vi "open_browser_send_url.vi"() -> ()   [LabVIEW 2018]
doc: "This VI uses ActiveX to open IE in its own window and point it to the URL typed into the string control."
panel:
  in  "Enter a URL and run the VI":string="http://192.168.169.3"
  in  "SHDocVw.IWebBrowser2":refnum<k7>
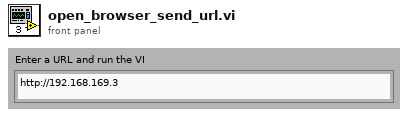
[diagram p1: front panel]
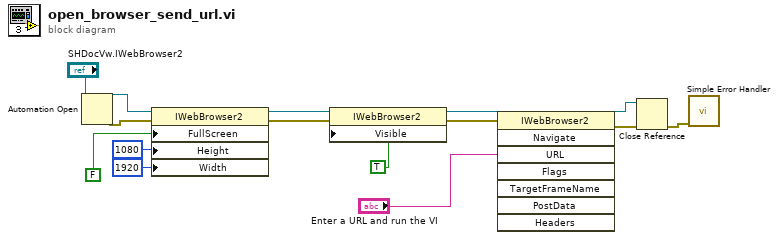
[diagram p0: block diagram]
diagram:
  n1 = Automation Open(Automation Refnum="SHDocVw.IWebBrowser2") -> (Automation Refnum=w15:refnum<k7>, error out=w14:errorcluster)  [unwired: 3 in]
  n2 = property class="IWebBrowser2"(reference=w15, error in=w14, "FullScreen"=FALSE, "Height"=1080, "Width"=1920) -> (reference out=w5:refnum<k7>, error out=w4:errorcluster)
  n3 = property class="IWebBrowser2"(reference=w5, error in=w4, "Visible"=TRUE) -> (reference out=w11:refnum<k7>, error out=w12:errorcluster)
  n4 = invoke class="IWebBrowser2" method="Navigate"(reference=w11, error in=w12, "URL"="Enter a URL and run the VI") -> (reference out=w8:refnum<k7>, error out=w9:errorcluster)  [unwired: 5 in, 6 out]
  n5 = Close Reference(reference=w8, error in (no error)=w9) -> (error out=w7:errorcluster)
  n6 = call <vilib>:"Simple Error Handler.vi"("error in (no error)"=w7) -> ()  [unwired: 4 in, 5 out]
